vi "dvr-redis-get.vi"(11 "redis-dvr":refnum<data-value>) -> (2 "Redis out":refnum<class "Redis.lvclass">)   [LabVIEW 2020, in "reporting-device.lvlib"]
uses:
  reporting-device.lvlib
  <userlib>/Zaphiro/GTools/Redis/Sources/Redis/Redis.lvclass
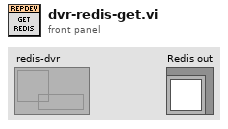
[diagram p1: front panel]
types:
  T1 = cluster{"output cluster":refnum<class "Redis.lvclass">}
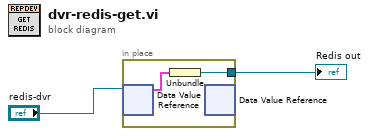
[diagram p0: block diagram]
diagram:
  n1 = in-place {
    in-place-border: [w3] -> w2
    n2 = in-place-dvr #1("redis-dvr") -> (w4:T1)  [unwired: 1 out]
    n3 = Unbundle(w4) -> ("output cluster"=w3:refnum<class "Redis.lvclass">)
    n4 = in-place-dvr #1() -> ()  [unwired: 1 in, 2 out]
  }
  "Redis out" <- w2
